vi "LDF Set Signal Value.vi"(7 "Value":dbl, 9 "pSignalName":string, 10 "pFrameName":string, 11 "LDFHandle":u64) -> (1 "pSignalName out":string, 2 "pFrameName out":string, 3 "function return":i32)   [LabVIEW 2010, in "ldf_parser.lvlib"]
doc: "int WINAPI LDF_SetSignalValue(long long LDFHandle, char* pFrameName, char* pSignalName, double Value);"
uses:
  ldf_parser.lvlib
  USB2XXX/trunk/USB2XXX/USB2XXX/vs2019/Release/USB2XXX.dll
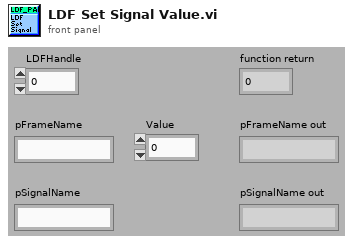
[diagram p1: front panel]
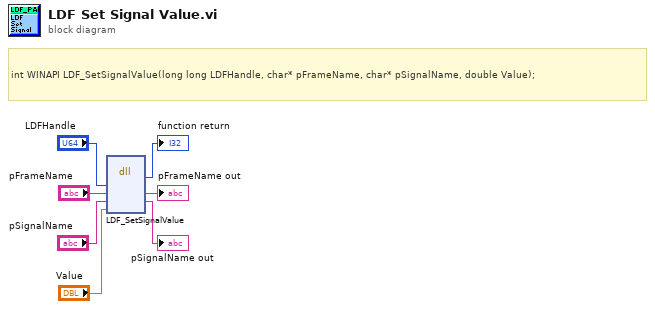
[diagram p0: block diagram]
diagram:
  # "int WINAPI LDF_SetSignalValue(long long LDFHandle, char* pFrameName, char* pSignalName, double Value);"
  n1 = dll-call lib="E:/Projects/USB2XXX/trunk/USB2XXX/USB2XXX/vs2019/Release/USB2XXX.*" fn="LDF_SetSignalValue"("LDFHandle"="LDFHandle", "pFrameName"="pFrameName", "pSignalName"="pSignalName", "Value"="Value") -> (→"function return":i32, "pFrameName"=→"pFrameName out":string, "pSignalName"=→"pSignalName out":string)  [unwired: 5 in, 2 out]
